vi "Read file configuration.vi"(8 "error in (no error)":errorcluster, 11 "Data Cluster":T1) -> (0 "error out":errorcluster, 3 "Data Cluster out":T1)   [LabVIEW 2020, in "Hardware DAQ.lvlib"]
uses:
  Hardware DAQ.lvlib
  Module Data--cluster.ctl
  <vilib>/Modbus/master/Modbus Master.lvclass
  <vilib>/Utility/config.llb/Read Key (String).vi
  <vilib>/Utility/config.llb/NI_LVConfig.lvlib
panel:
  out "string":string
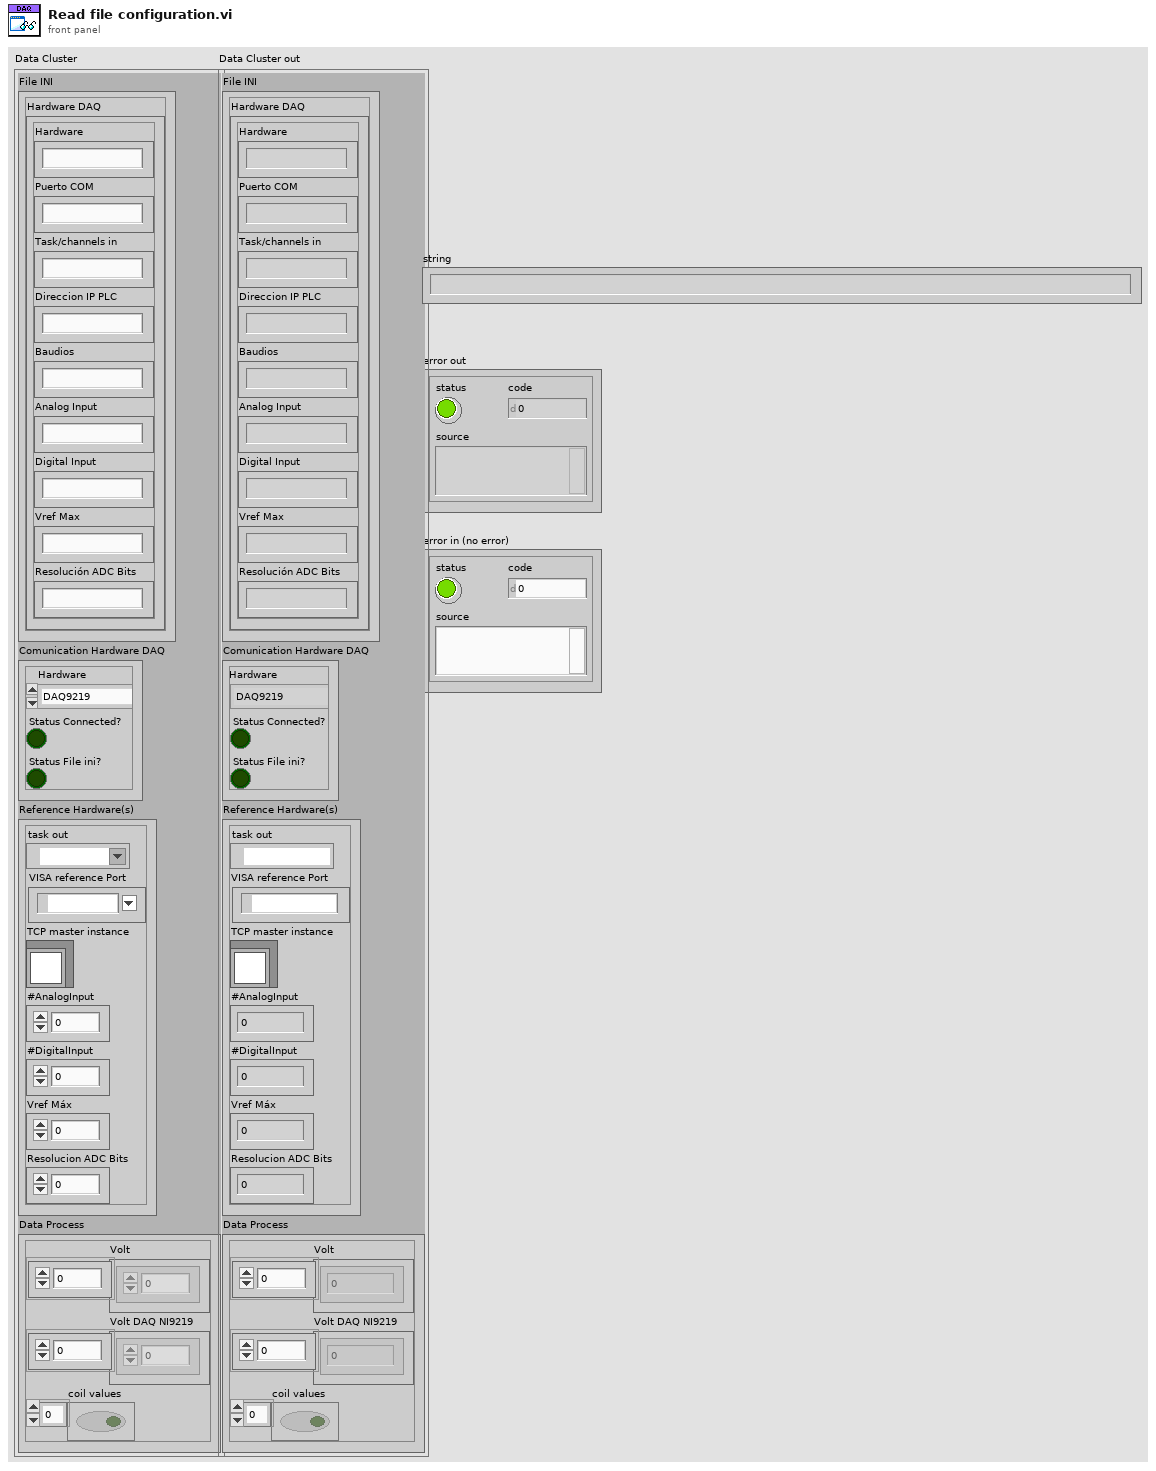
[diagram p1: front panel]
types:
  T1 = typedef "Hardware DAQ.lvlib/Module Data--cluster.ctl" = cluster{"File INI":cluster{"Hardware DAQ":cluster{"Hardware":string, "Puerto COM":string, "Task/channels in":string, "Direccion IP PLC":string, "Baudios":string, "Analog Input":string, "Digital Input":string, "Vref Max":string, "Resolución ADC Bits":string}}, "Comunication Hardware DAQ":cluster{"Hardware":enum16{"DAQ9219", "Arduino", "Xpress Board", "PLC Logo", "Default"}, "Status Connected?":bool, "Status File ini?":bool}, "Reference Hardware(s)":cluster{"task out":refnum<k21>, "VISA reference Port":refnum<visa-resource-name>, "TCP master instance":refnum<class "Modbus Master.lvclass">, "#AnalogInput":i32, "#DigitalInput":i32, "Vref Máx":i32, "Resolucion ADC Bits":i32}, "Data Process":cluster{"Volt":dbl[], "Volt DAQ NI9219":dbl[], "coil values":bool[]}}
  T2 = typedef "NI_LVConfig.lvlib/Config Data RefNum.ctl" = refnum<k1>
  T3 = cluster{"[0]":string, "[1]":string, "[2]":string, "[3]":string, "[4]":string, "[5]":string, "[6]":string, "[7]":string, "[8]":string}
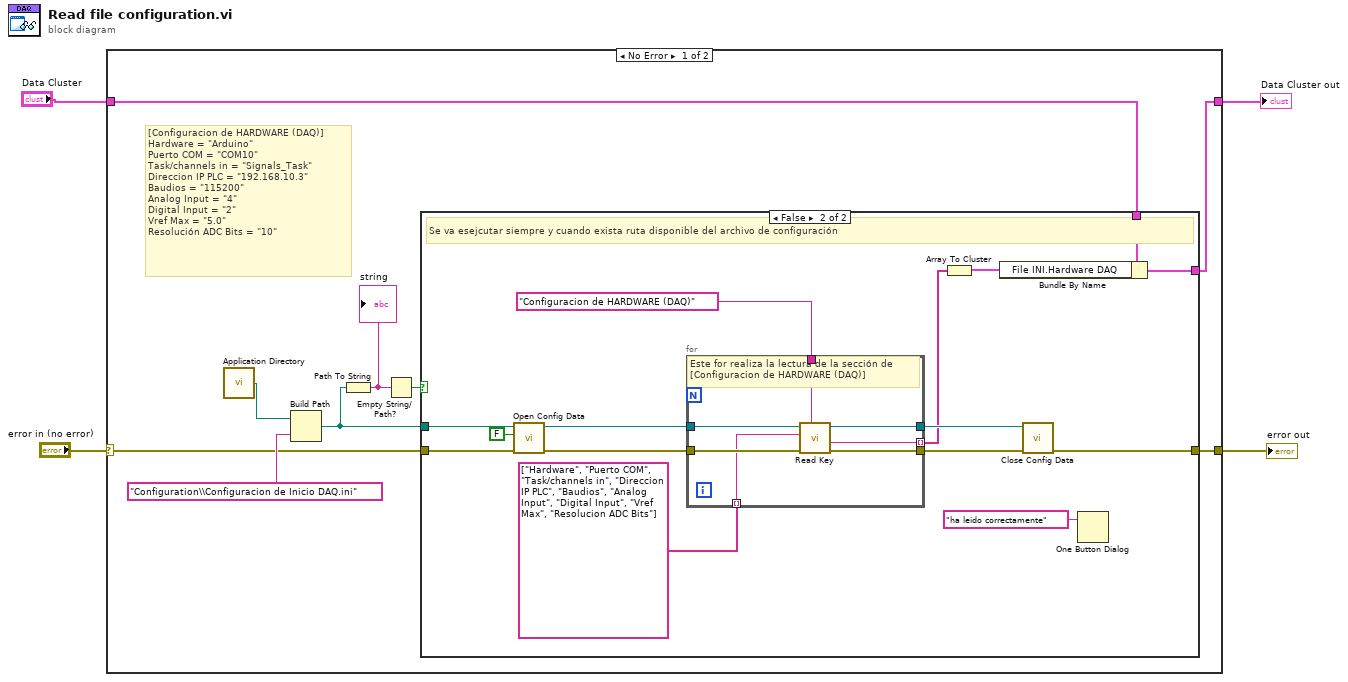
[diagram p0: block diagram]
diagram:
  n1 = case shown="No Error" "error in (no error)" {
    selector: "error in (no error)" -> [w11 w39]
    tunnel: [w10 w39] -> w4
    tunnel: "Data Cluster" -> [w9 w38]
    tunnel: [w8 w38] -> w1
    frame No Error {
      # "[Configuracion de HARDWARE (DAQ)]\nHardware = \"Arduino\"\nPuerto COM = \"COM10\"\nTask/channels in = \"Signals_Task\"\nDireccion IP PLC = \"192.168.10.3\"\nBaudios = \"115200\"\nAnalog Input = \"4\"\nDigital Input = \"2\"\nVref Max = \"5.0\"\nResolución ADC Bits = \"10\""
      n2 = call <vilib>:"Application Directory.vi"() -> ("Application Directory"=w12:path)
      n3 = Build Path(base path=w12, name or relative path="Configuration\\Configuracion de Inicio DAQ.ini") -> (appended path=w7:path)
      n4 = Path To String(path=w7) -> (string=w6:string)
      "string" <- w6
      n5 = Empty String/Path?(string/path=w6) -> (empty?=w5:bool)
      n6 = case shown="False" w5 {
        tunnel: w7 -> [_ w30]
        tunnel: w11 -> [w14 w29]
        tunnel: [w14 w18] -> w10
        tunnel: w9 -> [w15 w21]
        tunnel: [w15 w19] -> w8
        frame True {
        }
        frame False {
          # "Se va esejcutar siempre y cuando exista ruta disponible del archivo de configuración"
          n7 = call <vilib>:"Open Config Data.vi"("error in (no error)"=w29, "create file if necessary (T)"=FALSE, "configuration file path"=w30) -> ("error out"=w26:errorcluster, "refnum"=w27:T2)  [unwired: 6 in, 1 out]
          n8 = for {
            tunnel: w27 -> [w37]
            tunnel: w26 -> [w36]
            tunnel: [w35] -> w23
            tunnel: [w34] -> w24
            tunnel: "Configuracion de HARDWARE (DAQ)" -> [w33]
            tunnel: string[] ["Hardware", "Puerto COM", "Task/channels in", "Direccion IP PLC", "Baudios", "Analog Input", "Digital Input", "Vref Max", "Resolucion ADC Bits"] -> [w32] mode=indexing
            tunnel: [w31] -> w20 mode=indexing
            # "Este for realiza la lectura de la sección de\n[Configuracion de HARDWARE (DAQ)]"
            n9 = call-poly <vilib>:"Read Key.vi"("section"=w33, "error in (no error)"=w36, "key"=w32, "refnum"=w37) -> ("error out"=w35:errorcluster, "value"=w31:string, "refnum out"=w34:T2)  [unwired: 4 in, 1 out]
          }
          n10 = Array To Cluster(array=w20) -> (cluster=w17:T3)
          n11 = Bundle By Name(cluster=w21, "File INI.Hardware DAQ"=w17) -> (w19:T1)
          n12 = call <vilib>:"Close Config Data.vi"("error in (no error)"=w23, "refnum"=w24) -> ("error out"=w18:errorcluster)  [unwired: 8 in, 1 out]
          n13 = One Button Dialog(message="ha leido correctamente") -> ()  [unwired: 1 in, 1 out]
        }
      }
    }
    frame Error {
    }
  }
  "error out" <- w4
  "Data Cluster out" <- w1
